vi "Make AI JSON.vi"(9 "Force":bool, 10 "AI prev":T1={"type"="AI", "device"="", "name"="", "data"={"<init"=FALSE, "<avg_bits"=0, "<oversample_bits"=0, ">voltage"=0.0, " Accum Object"={"<init"=FALSE, ">value"=0.0, ">count"=0, "<center"=0, "<deadband"=0}}}, 11 "AI new":T1={"type"="AI", "device"="", "name"="", "data"={"<init"=FALSE, "<avg_bits"=0, "<oversample_bits"=0, ">voltage"=0.0, " Accum Object"={"<init"=FALSE, ">value"=0.0, ">count"=0, "<center"=0, "<deadband"=0}}}) -> (3 "delta JSON":string)   [LabVIEW 2019]
uses:
  AI proto.ctl
  AI Data proto.ctl
  AI Accum proto.ctl
panel:
  out "Complete JSON":string
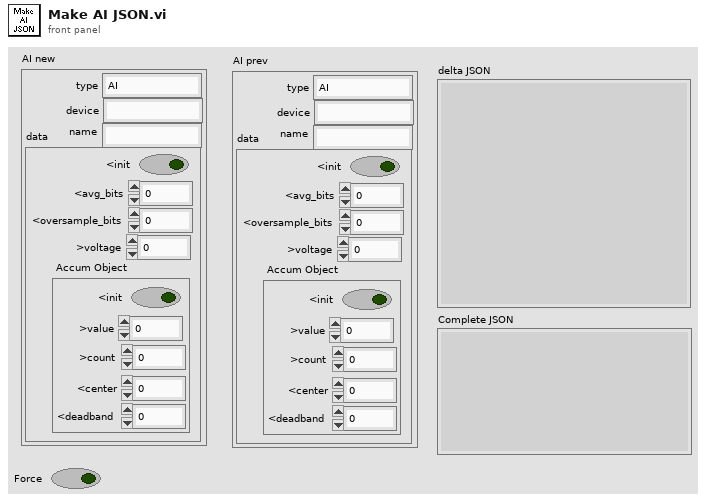
[diagram p1: front panel]
types:
  T1 = typedef "AI proto.ctl" = cluster{"type":string, "device":string, "name":string, "data":T2}
  T2 = typedef "AI Data proto.ctl" = cluster{"<init":bool, "<avg_bits":i32, "<oversample_bits":i32, ">voltage":dbl, " Accum Object":T3}
  T3 = typedef "AI Accum proto.ctl" = cluster{"<init":bool, ">value":dbl, ">count":i32, "<center":i32, "<deadband":i32}
  T4 = cluster{"type":bool, "device":bool, "name":bool, "data":cluster{"<init":bool, "<avg_bits":bool, "<oversample_bits":bool, ">voltage":bool, " Accum Object":cluster{"<init":bool, ">value":bool, ">count":bool, "<center":bool, "<deadband":bool}}}
  T5 = cluster{"<init":bool, "<avg_bits":bool, "<oversample_bits":bool, ">voltage":bool, " Accum Object":cluster{"<init":bool, ">value":bool, ">count":bool, "<center":bool, "<deadband":bool}}
  T6 = cluster{"<init":bool, ">value":bool, ">count":bool, "<center":bool, "<deadband":bool}
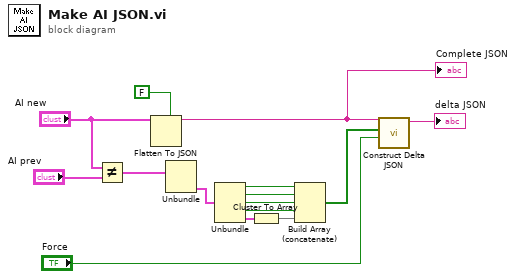
[diagram p0: block diagram]
diagram:
  n1 = Not Equal?(x="AI new", y="AI prev") -> (x != y?=w5:T4)
  n2 = Flatten To JSON(enable LabVIEW extensions? (T)=FALSE, anything="AI new") -> (JSON string=w4:string)  [unwired: 1 in, 1 out]
  "Complete JSON" <- w4
  n3 = Unbundle(w5) -> ("data"=w6:T5)  [unwired: 3 out]
  n4 = Unbundle(w6) -> ("<init"=w7:bool, "<avg_bits"=w8:bool, "<oversample_bits"=w9:bool, ">voltage"=w10:bool, "Accum Object"=w12:T6)
  n5 = Cluster To Array(cluster=w12) -> (array=w11:bool[])
  n6 = Build Array (concatenate)(w7, w8, w9, w10, w11) -> (w3:bool[])
  n7 = call "Construct Delta JSON.vi"("Force"="Force", "Checked Items"=w3, "JSON string"=w4) -> ("Delta JSON"=→"delta JSON":string)  [unwired: 8 in]
